vi "Extr patch AVIs paths.vi"(11 "ExperimentPath":path=path "D:/Srinivas/13 Patch Video/150610_14_10_33") -> (0 "error out":errorcluster, 2 "Extracted patches AVIs refs":T1[](array[typedef]), 3 "Extracted patches AVIs paths":path[](array[path]))   [LabVIEW 2017]
uses:
  <vilib>/vision/Avi.llb/IMAQ AVI2 Refnum.ctl
  <userlib>/_OpenG.lib/array/array.llb/Sort 1D Array (String)__ogtk.vi
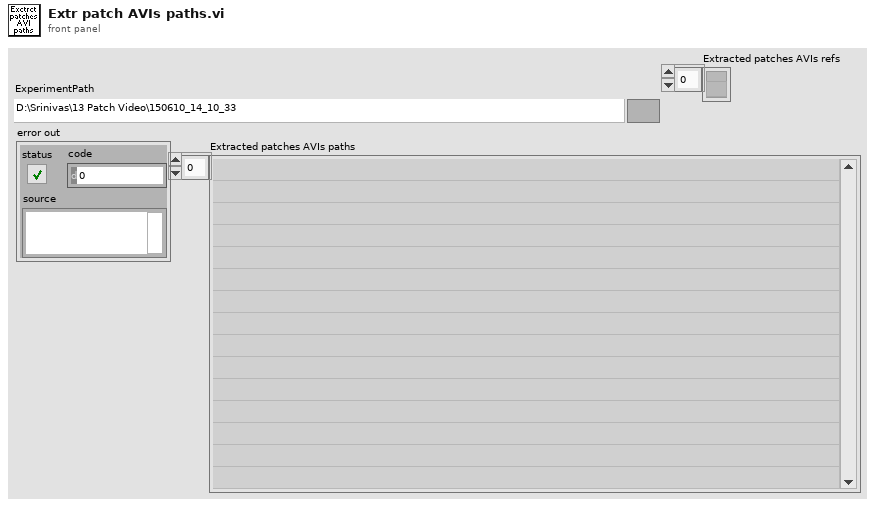
[diagram p1: front panel]
types:
  T1 = typedef "IMAQ AVI2 Refnum.ctl" = refnum<k20>
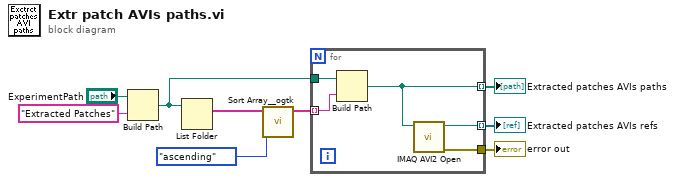
[diagram p0: block diagram]
diagram:
  n1 = Build Path(base path="ExperimentPath", name or relative path="Extracted Patches") -> (appended path=w7:path)
  n2 = List Folder(path=w7) -> (filenames=w5:string[])  [unwired: 3 in, 3 out]
  n3 = call-poly <userlib>:"Sort Array__ogtk.vi"("Order"=enum16{"ascending", "descending"}."ascending", "Array in"=w5) -> ("Sorted Array out"=w4:string[])  [unwired: 8 in, 1 out]
  n4 = for {
    tunnel: w7 -> [w14]
    tunnel: w4 -> [w13] mode=indexing
    tunnel: [w12] -> w6 mode=indexing
    tunnel: [w11] -> w2 mode=indexing
    tunnel: [w10] -> w1
    n5 = Build Path(base path=w14, name or relative path=w13) -> (appended path=w12:path)
    n6 = call "IMAQ AVI2 Open"("AVI File Path"=w12) -> ("error out"=w10:errorcluster, "AVI Refnum"=w11:T1)  [unwired: 9 in]
  }
  "Extracted patches AVIs paths" <- w6
  "Extracted patches AVIs refs" <- w2
  "error out" <- w1
